vi "importLiquidDelivery.vi"(8 "error in (no error)":errorcluster, 10 "Tuple":T1={"mouse_id"=1217.0, "session_timestamp"="", "timestamp"=0.0, "pulse_time"=0.0, "microl_per_pulse"=0.0, "liquid_type"=""}, 11 "Database in":refnum<class "Database.lvclass">) -> (0 "error out":errorcluster, 3 "Database out":refnum<class "Database.lvclass">)   [LabVIEW 2014, in "Database.lvclass"]
uses:
  Database.lvclass
  Database.lvclass/Database.ctl
  <vilib>/addons/database/NI_Database_API.lvlib
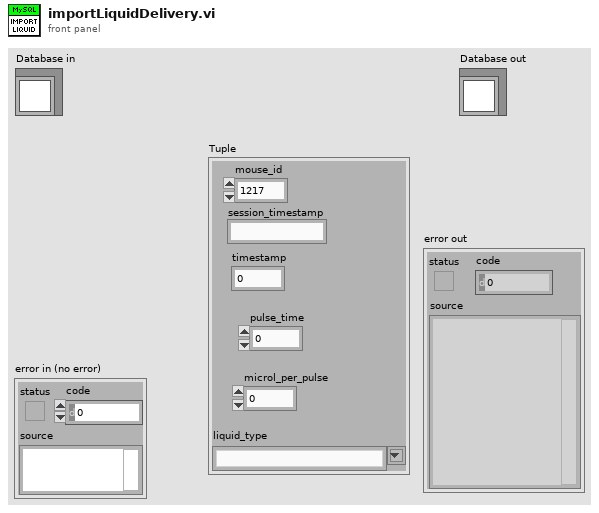
[diagram p1: front panel]
types:
  T1 = cluster{"mouse_id":dbl, "session_timestamp":string, "timestamp":dbl, "pulse_time":dbl, "microl_per_pulse":dbl, "liquid_type":string}
  T2 = typedef "NI_Database_API.lvlib/Conn ObjectReference.ctl" = refnum<k1>
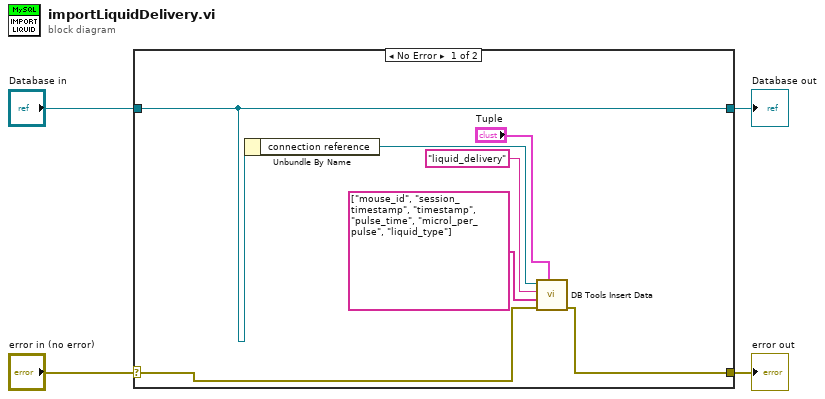
[diagram p0: block diagram]
diagram:
  n1 = case shown="No Error" "error in (no error)" {
    selector: "error in (no error)" -> [w7 w13]
    tunnel: [w6 w13] -> w3
    tunnel: [w5 w12] -> w1
    tunnel: "Database in" -> [w5 w12]
    frame No Error {
      n2 = Unbundle By Name(w5) -> ("connection reference"=w9:T2)
      n3 = call <vilib>:"DB Tools Insert Data.vi"("data"="Tuple", "error in (no error)"=w7, "columns"=string[] ["mouse_id", "session_timestamp", "timestamp", "pulse_time", "microl_per_pulse", "liquid_type"], "table"="liquid_delivery", "connection reference"=w9) -> ("error out"=w6:errorcluster)  [unwired: 5 in, 1 out]
    }
    frame Error {
    }
  }
  "error out" <- w3
  "Database out" <- w1
